vi "Lift.vi"(0 "LiftLocation":T1(ring)) -> ()   [LabVIEW 2018]
uses:
  <vilib>/Rock Robotics/SystemInterfaces/DIO/FPGA_DIOChannel.ctl
  <vilib>/Rock Robotics/WPI/ThirdParty/Phoenix-LabVIEW/Motor Controller/Controls/CTRE_Phoenix_MotorControl_ControlMode.ctl
  Lift Global.vi
  Times/Times Global.vi
  <vilib>/addons/control/pid/pid.llb/PID (DBL).vi
  <vilib>/Rock Robotics/WPI/ThirdParty/Phoenix-LabVIEW/Motor Controller/Get/CTRE_Phoenix_MotorController_GetSelectedSensorData.vi
  Cargo Intake/Cargo Intake Global.vi
  <vilib>/addons/control/pid/NI_PID_pid.lvlib
panel:
  in  "Output Scalar":dbl=0.8 format="%#_13g"
  in  "t":dbl=0.5 format="%#_13g"
  in  "output range":cluster{"output high":dbl, "output low":dbl}={"output high"=1.0, "output low"=-0.5}
  in  "LiftMode":T2(ring)=enum."Basic Control"
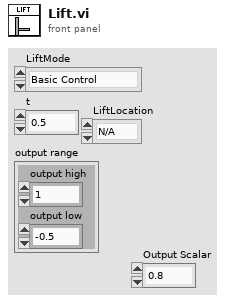
[diagram p1: front panel]
types:
  T1 = enum16{"N/A", "Hatch Panel Zone 1", "Hatch Panel Zone 2", "Hatch Panel Zone 3", "Cargo Zone 1", "Cargo Zone 2", "Cargo Zone 3"}
  T2 = enum16{"Ultra Manual Control", "Manual Control", "Basic Control", "Automated Control", "Autonomous Control"}
  T3 = typedef "FPGA_DIOChannel.ctl" = enum8{"DIO 0", "DIO 1", "DIO 2", "DIO 3", "DIO 4", "DIO 5", "DIO 6", "DIO 7", "DIO 8", "DIO 9", "DIO MXP 0", "DIO MXP 1", "DIO MXP 2", "DIO MXP 3", "DIO MXP 4", "DIO MXP 5", "DIO MXP 6", "DIO MXP 7", "DIO MXP 8", "DIO MXP 9", "DIO MXP 10", "DIO MXP 11", "DIO MXP 12", "DIO MXP 13", "DIO MXP 14", "DIO MXP 15", "SPI Port CS1", "SPI Port CS2", "SPI Port CS3", "SPI Port MISO", "SPI Port MOSI", "Invalid"}
  T4 = typedef "WPI_MotorControlDeviceRef.ctl" = cluster{"DeviceStatus":errorcluster, "Type":T5, "PWM":cluster{"PWM Channel":T6, "DeadBand":T7}, "CAN":cluster{"Device Number":u8, "SetOutput VI Ref":variant, "GetOutput VI Ref":variant, "Enable VI Ref":variant, "Disable VI Ref":variant, "Data":variant}, "Invert":bool, "DIO PWM":cluster{"PWM \"Enable\" Channel":T6, "DIOChannel":T3, "PWM Rate":dbl}}
  T5 = typedef "WPI_MotorControlType.ctl" = enum16{"PWM", "CAN", "DIO PWM"}
  T6 = typedef "FPGA_DIOPWMChannel.ctl" = enum8{"PWM 0", "PWM 1", "PWM 2", "PWM 3", "PWM 4", "PWM 5", "PWM 6", "PWM 7", "PWM 8", "PWM 9", "PWM MXP 0", "PWM MXP 1", "PWM MXP 2", "PWM MXP 3", "PWM MXP 4", "PWM MXP 5", "PWM MXP 6", "PWM MXP 7", "PWM MXP 8", "PWM MXP 9", "Invalid"}
  T7 = typedef "WPI_PWMDeadband.ctl" = cluster{"Name":string, "maxPositivePwm":i32, "minPositivePwm":i32, "centerPwm":i32, "maxNegativePwm":i32, "minNegativePwm":i32, "angularRange":u16}
  T8 = typedef "WPI_DigitalInputDevRef.ctl" = cluster{"DevStatus":errorcluster, "DIO Channel":T3}
  T9 = typedef "CTRE_Phoenix_MotorControl_ControlMode.ctl" = u16
  T10 = cluster{"proportional gain (Kc)":dbl, "integral time(Ti, min)":dbl, "derivative time(Td, min) 2":dbl}
  T11 = enum16{"Hatch Panel Zone 1", "Hatch Panel Zone 2", "Hatch Panel Zone 3", "Cargo Zone 1", "Cargo Zone 2", "Cargo Zone 3", "Cargo Ship Zone"}
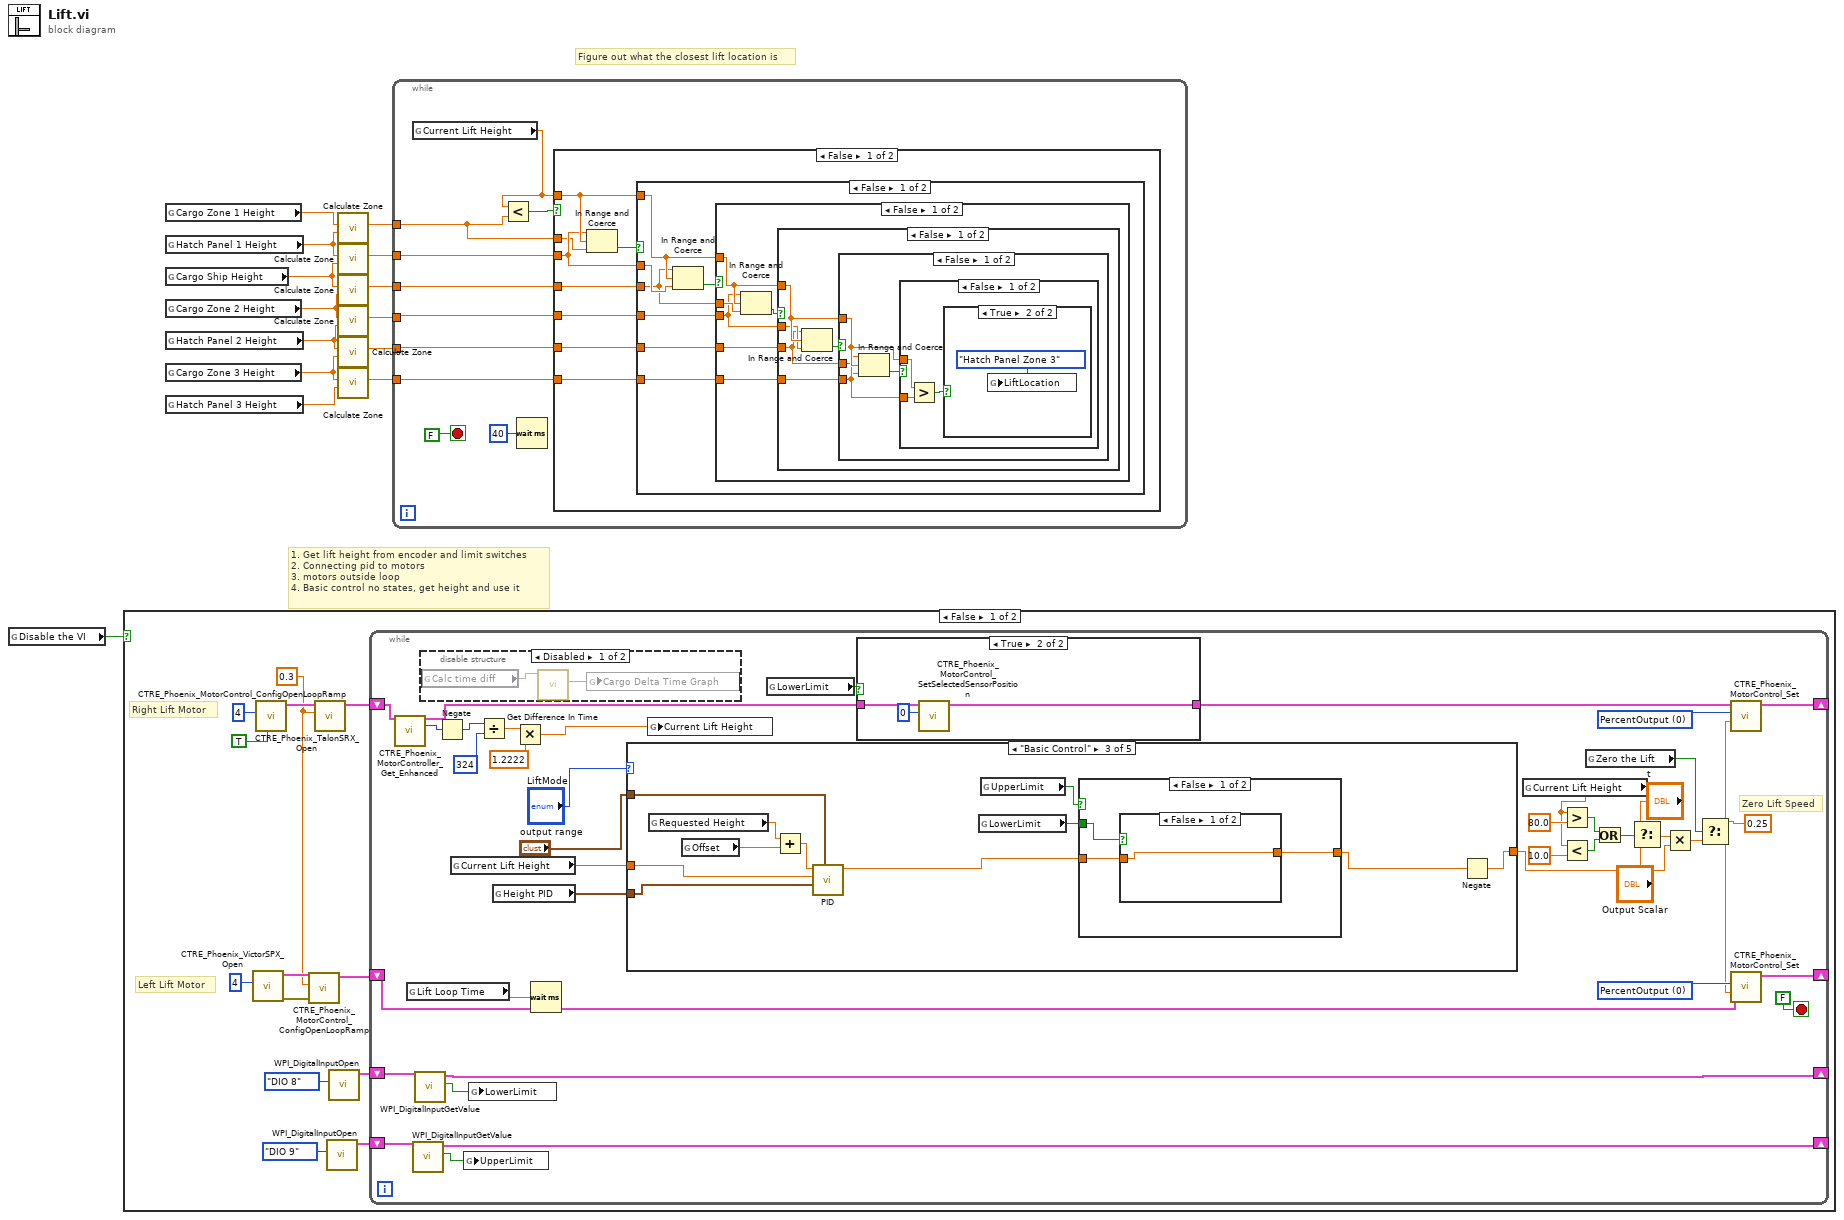
[diagram p0: block diagram]
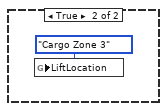
[diagram p3: hidden frame]
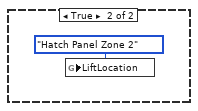
[diagram p4: hidden frame]
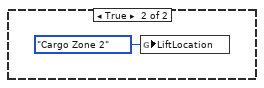
[diagram p5: hidden frame]
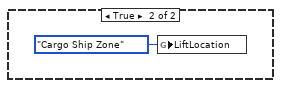
[diagram p6: hidden frame]
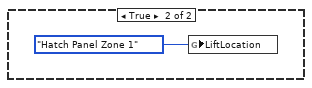
[diagram p7: hidden frame]
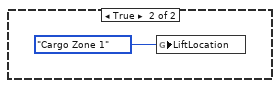
[diagram p8: hidden frame]
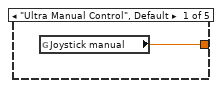
[diagram p11: hidden frame]
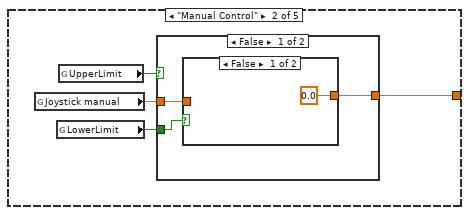
[diagram p12: hidden frame]
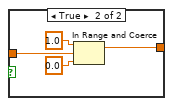
[diagram p13: hidden frame]
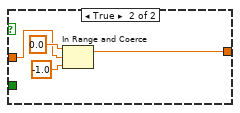
[diagram p14: hidden frame]
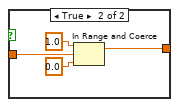
[diagram p15: hidden frame]
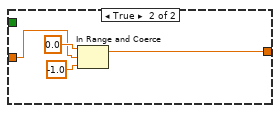
[diagram p16: hidden frame]
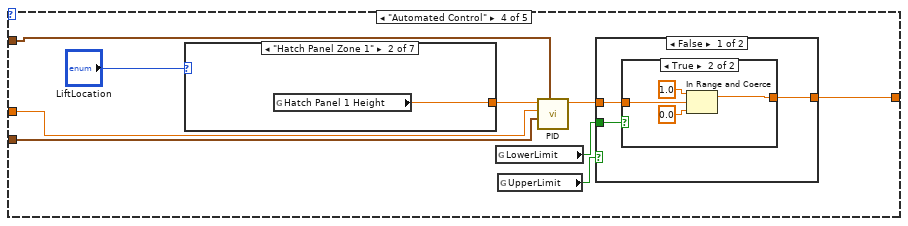
[diagram p17: hidden frame]
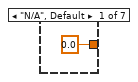
[diagram p18: hidden frame]
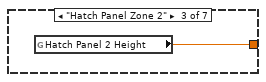
[diagram p19: hidden frame]
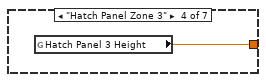
[diagram p20: hidden frame]
diagram:
  # "Figure out what the closest lift location is"
  # "1. Get lift height from encoder and limit switches\n2. Connecting pid to motors\n3. motors outside loop\n4. Basic control no states, get height and use it"
  n1 = global read "Lift Global.vi" "Disable the VI"() -> (w14:bool)
  n2 = case shown="False" w14 {
    frame False {
      w16 = 0.3 ("secondsFromNeutralToFull")
      # "Left Lift Motor"
      # "Right Lift Motor"
      n3 = call <vilib>:"CTRE_Phoenix_VictorSPX_Open.vi"("Device Number"=u8 4) -> ("error out"=w19:errorcluster, "CAN Talon SRX Ref"=w18:T4)  [unwired: 9 in]
      n4 = call <vilib>:"CTRE_Phoenix_TalonSRX_Open.vi"("Invert"=TRUE, "Device Number"=u8 4) -> ("CAN Talon SRX Ref"=w21:T4)  [unwired: 8 in, 1 out]
      n5 = call <vilib>:"CTRE_Phoenix_MotorControl_ConfigOpenLoopRamp.vi"("error in (no error)"=w19, "secondsFromNeutralToFull"=w16, "PhoenixMotorControlDevRef"=w18) -> ("PhoenixMotorControlDevRef"=w17:T4)  [unwired: 7 in, 1 out]
      n6 = call <vilib>:"CTRE_Phoenix_MotorControl_ConfigOpenLoopRamp.vi"("secondsFromNeutralToFull"=w16, "PhoenixMotorControlDevRef"=w21) -> ("PhoenixMotorControlDevRef"=w20:T4)  [unwired: 8 in, 1 out]
      n7 = call <vilib>:"WPI_DigitalInputOpen.vi"("DIO Channel"=FPGA_DIOChannel."DIO 9") -> ("DigitalInputDevRef"=w22:T8)  [unwired: 9 in, 1 out]
      n8 = call <vilib>:"WPI_DigitalInputOpen.vi"("DIO Channel"=FPGA_DIOChannel."DIO 8") -> ("DigitalInputDevRef"=w24:T8)  [unwired: 9 in, 1 out]
      n9 = while {
        shift-right: [w64] -> _
        shift-left: w20 -> [w57]
        shift-right: [w62] -> _
        shift-left: w17 -> [w61]
        shift-right: [w52] -> _
        shift-left: w24 -> [w53]
        shift-right: [w47] -> _
        shift-left: w22 -> [w48]
        stop <- FALSE stop-if-true
        w63 = T9 0 items=["PercentOutput"=0, "Position"=1, "Velocity"=2, "Current"=3, "Follower"=5, "MotionProfile"=6, "MotionMagic"=7, "MotionProfileArc"=10, "Disabled"=15] ("Control Mode")
        w65 = T9 0 items=["PercentOutput"=0, "Position"=1, "Velocity"=2, "Current"=3, "Follower"=5, "MotionProfile"=6, "MotionMagic"=7, "MotionProfileArc"=10, "Disabled"=15] ("Control Mode")
        # "Zero Lift Speed"
        n10 = call-poly <vilib>:"CTRE_Phoenix_MotorController_Get_Enhanced.vi"("PhoenixMotorControlDevRef"=w57) -> ("PhoenixMotorControlDevRef"=w56:T4, "Position (Raw Sensor Units)"=w28:i32)  [unwired: 11 in, 2 out]
        n11 = global read "Times Global.vi" "Lift Loop Time"() -> (w68:dbl)
        n12 = call <vilib>:"WPI_DigitalInputGetValue.vi"("DigitalInputDevRef"=w48) -> ("Value"=w50:bool, "DigitalInputDevRef"=w47:T8)  [unwired: 8 in, 1 out]
        n13 = call <vilib>:"WPI_DigitalInputGetValue.vi"("DigitalInputDevRef"=w53) -> ("Value"=w51:bool, "DigitalInputDevRef"=w52:T8)  [unwired: 8 in, 1 out]
        n14 = disable-structure shown="Disabled" {
          frame Disabled {
            n15 = global read "Cargo Intake Global.vi" "Calc time diff"() -> (w74:bool)
            n16 = call "Get Difference In Time.vi"("Calculate Time Difference"=w74) -> ("Delta Time over Time"=w73:u32)  [unwired: 9 in, 1 out]
            n17 = global write "Times Global.vi" "Cargo Delta Time Graph"(w73) -> ()
          }
          frame Enabled {
          }
        }
        n18 = Negate(x=w28) -> (-x=w29:i32)
        n19 = global read "Lift Global.vi" "Current Lift Height"() -> (w58:dbl)
        n20 = global write "Lift Global.vi" "UpperLimit"(w50) -> ()
        n21 = global write "Lift Global.vi" "LowerLimit"(w51) -> ()
        n22 = Divide(x=w29, y=324) -> (x/y=w36:dbl)
        n23 = global read "Lift Global.vi" "Height PID"() -> (w59:T10)
        n24 = Multiply(x=w36, y=1.2222) -> (x*y=w34:dbl)
        n25 = Wait (ms)(milliseconds to wait=w68) -> ()  [unwired: 1 out]
        n26 = case shown="\"Basic Control\"" "LiftMode" {
          tunnel: [w75 w76 w99 w120 0.0 ("Cargo Zone 3 Height")] -> w39
          tunnel: w58 -> [_ _ w102 w118 _]
          tunnel: w59 -> [_ _ w101 w117 _]
          tunnel: "output range" -> [_ _ w100 w119 _]
          frame "Ultra Manual Control", Default {
            n27 = global read "Lift Global.vi" "Joystick manual"() -> (w75:dbl)
          }
          frame "Manual Control" {
            n28 = global read "Lift Global.vi" "Joystick manual"() -> (w77:dbl)
            n29 = global read "Lift Global.vi" "LowerLimit"() -> (w79:bool)
            n30 = global read "Lift Global.vi" "UpperLimit"() -> (w78:bool)
            n31 = case shown="False" w78 {
              tunnel: w79 -> [w82 _]
              tunnel: [w81 w89] -> w76
              tunnel: w77 -> [w80 w88]
              frame False {
                n32 = case shown="False" w82 {
                  tunnel: [0.0 w87] -> w81
                  tunnel: w80 -> [_ w84]
                  frame False {
                  }
                  frame True {
                    n33 = In Range and Coerce(upper limit=1.0, x=w84, lower limit=0.0) -> (coerced(x)=w87:dbl)  [unwired: 1 out]
                  }
                }
              }
              frame True {
                n34 = In Range and Coerce(upper limit=0.0, x=w88, lower limit=-1.0) -> (coerced(x)=w89:dbl)  [unwired: 1 out]
              }
            }
          }
          frame "Basic Control" {
            n35 = global read "Lift Global.vi" "Requested Height"() -> (w92:dbl)
            n36 = global read "Lift Global.vi" "Offset"() -> (w93:dbl)
            n37 = Add(x=w92, y=w93) -> (x+y=w94:dbl)
            n38 = call-poly <vilib>:"PID.vi"("output range"=w100, "PID gains"=w101, "process variable"=w102, "setpoint"=w94) -> ("output"=w96:dbl)  [unwired: 6 in, 1 out]
            n39 = global read "Lift Global.vi" "LowerLimit"() -> (w98:bool)
            n40 = global read "Lift Global.vi" "UpperLimit"() -> (w97:bool)
            n41 = case shown="False" w97 {
              tunnel: w98 -> [w105 _]
              tunnel: [w104 w112] -> w95
              tunnel: w96 -> [w103 w111]
              frame False {
                n42 = case shown="False" w105 {
                  tunnel: [w106 w110] -> w104
                  tunnel: w103 -> [w106 w107]
                  frame False {
                  }
                  frame True {
                    n43 = In Range and Coerce(upper limit=1.0, x=w107, lower limit=0.0) -> (coerced(x)=w110:dbl)  [unwired: 1 out]
                  }
                }
              }
              frame True {
                n44 = In Range and Coerce(upper limit=0.0, x=w111, lower limit=-1.0) -> (coerced(x)=w112:dbl)  [unwired: 1 out]
              }
            }
            n45 = Negate(x=w95) -> (-x=w99:dbl)
          }
          frame "Automated Control" {
            n46 = case shown="\"Hatch Panel Zone 1\"" "LiftLocation" {
              tunnel: [0.0 ("Cargo Zone 3 Height") w125 w126 w127 w128 w129 w130] -> w115
              frame "N/A", Default {
              }
              frame "Hatch Panel Zone 1" {
                n47 = global read "Lift Global.vi" "Hatch Panel 1 Height"() -> (w125:dbl)
              }
              frame "Hatch Panel Zone 2" {
                n48 = global read "Lift Global.vi" "Hatch Panel 2 Height"() -> (w126:dbl)
              }
              frame "Hatch Panel Zone 3" {
                n49 = global read "Lift Global.vi" "Hatch Panel 3 Height"() -> (w127:dbl)
              }
              frame "Cargo Zone 1" {
                n50 = global read "Lift Global.vi" "Cargo Zone 1 Height"() -> (w128:dbl)
              }
              frame "Cargo Zone 2" {
                n51 = global read "Lift Global.vi" "Cargo Zone 2 Height"() -> (w129:dbl)
              }
              frame "Cargo Zone 3" {
                n52 = global read "Lift Global.vi" "Cargo Zone 3 Height"() -> (w130:dbl)
              }
            }
            n53 = global read "Lift Global.vi" "LowerLimit"() -> (w123:bool)
            n54 = global read "Lift Global.vi" "UpperLimit"() -> (w122:bool)
            n55 = call-poly <vilib>:"PID.vi"("output range"=w119, "PID gains"=w117, "process variable"=w118, "setpoint"=w115) -> ("output"=w121:dbl)  [unwired: 6 in, 1 out]
            n56 = case shown="False" w122 {
              tunnel: w123 -> [w133 _]
              tunnel: [w132 w140] -> w120
              tunnel: w121 -> [w131 w139]
              frame False {
                n57 = case shown="True" w133 {
                  tunnel: [0.0 w138] -> w132
                  tunnel: w131 -> [_ w135]
                  frame False {
                  }
                  frame True {
                    n58 = In Range and Coerce(upper limit=1.0, x=w135, lower limit=0.0) -> (coerced(x)=w138:dbl)  [unwired: 1 out]
                  }
                }
              }
              frame True {
                n59 = In Range and Coerce(upper limit=0.0, x=w139, lower limit=-1.0) -> (coerced(x)=w140:dbl)  [unwired: 1 out]
              }
            }
          }
          frame "Autonomous Control" {
          }
        }
        n60 = global write "Lift Global.vi" "Current Lift Height"(w34) -> ()
        n61 = global read "Lift Global.vi" "LowerLimit"() -> (w49:bool)
        n62 = case shown="True" w49 {
          tunnel: w56 -> [w69 w72]
          tunnel: [w69 w71] -> w55
          frame False {
          }
          frame True {
            n63 = call <vilib>:"CTRE_Phoenix_MotorControl_SetSelectedSensorPosition.vi"("New Sensor Position"=0, "PhoenixMotorControlDevRef"=w72) -> ("PhoenixMotorControlDevRef"=w71:T4)  [unwired: 8 in, 1 out]
          }
        }
        n64 = global read "Lift Global.vi" "Current Lift Height"() -> (w44:dbl)
        n65 = Greater?(x=w44, y=80.0) -> (0:w42:bool)
        n66 = Less?(x=w44, y=10.0) -> (x < y?=w43:bool)
        n67 = global read "Lift Global.vi" "Zero the Lift"() -> (w32:bool)
        n68 = Or(x=w42, y=w43) -> (x .or. y?=w41:bool)
        n69 = Select(t="t", s=w41, f="Output Scalar") -> (s? t:f=w40:dbl)
        n70 = Multiply(x=w40, y=w39) -> (x*y=w33:dbl)
        n71 = Select(t=0.25, s=w32, f=w33) -> (s? t:f=w30:dbl)
        n72 = call <vilib>:"CTRE_Phoenix_MotorControl_Set.vi"("Output"=w30, "Control Mode"=w65, "PhoenixMotorControlDevRef"=w55) -> ("PhoenixMotorControlDevRef"=w64:T4)  [unwired: 7 in, 1 out]
        n73 = call <vilib>:"CTRE_Phoenix_MotorControl_Set.vi"("Output"=w30, "Control Mode"=w63, "PhoenixMotorControlDevRef"=w61) -> ("PhoenixMotorControlDevRef"=w62:T4)  [unwired: 7 in, 1 out]
      }
    }
    frame True {
    }
  }
  n74 = global read "Lift Global.vi" "Cargo Zone 1 Height"() -> (w7:dbl)
  n75 = global read "Lift Global.vi" "Hatch Panel 1 Height"() -> (w13:dbl)
  n76 = global read "Lift Global.vi" "Cargo Ship Height"() -> (w12:dbl)
  n77 = global read "Lift Global.vi" "Cargo Zone 2 Height"() -> (w11:dbl)
  n78 = global read "Lift Global.vi" "Hatch Panel 2 Height"() -> (w10:dbl)
  n79 = global read "Lift Global.vi" "Cargo Zone 3 Height"() -> (w9:dbl)
  n80 = global read "Lift Global.vi" "Hatch Panel 3 Height"() -> (w8:dbl)
  n81 = call "Calculate Zone.vi"("Top Height"=w13, "Bottom Height"=w7) -> ("Midpoint"=w6:dbl)  [unwired: 9 in]
  n82 = call "Calculate Zone.vi"("Top Height"=w12, "Bottom Height"=w13) -> ("Midpoint"=w5:dbl)  [unwired: 9 in]
  n83 = call "Calculate Zone.vi"("Top Height"=w11, "Bottom Height"=w12) -> ("Midpoint"=w4:dbl)  [unwired: 9 in]
  n84 = call "Calculate Zone.vi"("Top Height"=w10, "Bottom Height"=w11) -> ("Midpoint"=w3:dbl)  [unwired: 9 in]
  n85 = call "Calculate Zone.vi"("Top Height"=w9, "Bottom Height"=w10) -> ("Midpoint"=w2:dbl)  [unwired: 9 in]
  n86 = call "Calculate Zone.vi"("Top Height"=w8, "Bottom Height"=w9) -> ("Midpoint"=w1:dbl)  [unwired: 9 in]
  n87 = while {
    tunnel: w6 -> [w149]
    tunnel: w5 -> [w148]
    tunnel: w4 -> [w147]
    tunnel: w3 -> [w146]
    tunnel: w2 -> [w145]
    tunnel: w1 -> [w144]
    stop <- FALSE stop-if-true
    n88 = global read "Lift Global.vi" "Current Lift Height"() -> (w150:dbl)
    n89 = Less?(x=w150, y=w149) -> (x < y?=w151:bool)
    n90 = Wait (ms)(milliseconds to wait=u32 40) -> ()  [unwired: 1 out]
    n91 = case shown="False" w151 {
      tunnel: w150 -> [w157 _]
      tunnel: w149 -> [w155 _]
      tunnel: w148 -> [w156 _]
      tunnel: w147 -> [w161 _]
      tunnel: w146 -> [w160 _]
      tunnel: w145 -> [w159 _]
      tunnel: w144 -> [w158 _]
      frame False {
        n92 = In Range and Coerce(upper limit=w156, x=w157, lower limit=w155) -> (In Range?=w154:bool)  [unwired: 1 out]
        n93 = case shown="False" w154 {
          tunnel: w157 -> [w164 _]
          tunnel: w156 -> [w163 _]
          tunnel: w161 -> [w162 _]
          tunnel: w160 -> [w168 _]
          tunnel: w159 -> [w167 _]
          tunnel: w158 -> [w166 _]
          frame False {
            n94 = In Range and Coerce(upper limit=w162, x=w164, lower limit=w163) -> (In Range?=w165:bool)  [unwired: 1 out]
            n95 = case shown="False" w165 {
              tunnel: w164 -> [w171 _]
              tunnel: w168 -> [w169 _]
              tunnel: w167 -> [w174 _]
              tunnel: w166 -> [w173 _]
              tunnel: w162 -> [w170 _]
              frame False {
                n96 = In Range and Coerce(upper limit=w169, x=w171, lower limit=w170) -> (In Range?=w172:bool)  [unwired: 1 out]
                n97 = case shown="False" w172 {
                  tunnel: w171 -> [w177 _]
                  tunnel: w174 -> [w175 _]
                  tunnel: w173 -> [w179 _]
                  tunnel: w169 -> [w176 _]
                  frame False {
                    n98 = In Range and Coerce(upper limit=w175, x=w177, lower limit=w176) -> (In Range?=w178:bool)  [unwired: 1 out]
                    n99 = case shown="False" w178 {
                      tunnel: w177 -> [w182 _]
                      tunnel: w179 -> [w181 _]
                      tunnel: w175 -> [w180 _]
                      frame False {
                        n100 = In Range and Coerce(upper limit=w181, x=w182, lower limit=w180) -> (In Range?=w183:bool)  [unwired: 1 out]
                        n101 = case shown="False" w183 {
                          tunnel: w182 -> [w186 _]
                          tunnel: w181 -> [w185 _]
                          frame False {
                            n102 = Greater?(x=w186, y=w185) -> (0:w184:bool)
                            n103 = case shown="True" w184 {
                              frame False {
                              }
                              frame True {
                                n104 = global write "Lift Global.vi" "LiftLocation"(T11."Hatch Panel Zone 3" ("LiftLocation")) -> ()
                              }
                            }
                          }
                          frame True {
                            n105 = global write "Lift Global.vi" "LiftLocation"(T11."Cargo Zone 3" ("LiftLocation")) -> ()
                          }
                        }
                      }
                      frame True {
                        n106 = global write "Lift Global.vi" "LiftLocation"(T11."Hatch Panel Zone 2" ("LiftLocation")) -> ()
                      }
                    }
                  }
                  frame True {
                    n107 = global write "Lift Global.vi" "LiftLocation"(T11."Cargo Zone 2" ("LiftLocation")) -> ()
                  }
                }
              }
              frame True {
                n108 = global write "Lift Global.vi" "LiftLocation"(T11."Cargo Ship Zone" ("LiftLocation")) -> ()
              }
            }
          }
          frame True {
            n109 = global write "Lift Global.vi" "LiftLocation"(T11."Hatch Panel Zone 1" ("LiftLocation")) -> ()
          }
        }
      }
      frame True {
        n110 = global write "Lift Global.vi" "LiftLocation"(T11."Cargo Zone 1" ("LiftLocation")) -> ()
      }
    }
  }
